vi "Destroy.vi"(8 "ErrorIn":errorcluster, 11 "ReferenceIn":refnum<class "VerticalButtonBar.lvclass">) -> (0 "ErrorOut":errorcluster, 3 "ReferenceOut":refnum<class "VerticalButtonBar.lvclass">)   [LabVIEW 2021, in "VerticalButtonBar.lvclass"]
doc: "Destroy the object instance"
uses:
  VerticalButtonBar.lvclass
  .Externals/Library_TAF_ApplicationFramework/TAFBaseGUI/TAFBaseGUI.lvclass
  VerticalButtonBar.lvclass/VerticalButtonBar.ctl
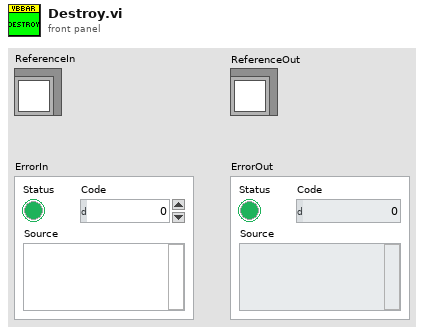
[diagram p1: front panel]
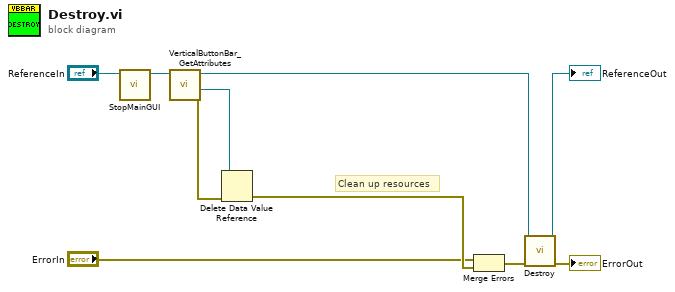
[diagram p0: block diagram]
diagram:
  # "Clean up resources"
  n1 = call "StopMainGUI.vi"("ReferenceIn"="ReferenceIn") -> ("ReferenceOut"=w3:refnum<class "VerticalButtonBar.lvclass">)  [unwired: 9 in, 1 out]
  n2 = call "VerticalButtonBar_GetAttributes.vi"("ReferenceIn"=w3) -> ("ErrorOut"=w10:errorcluster, "DataRef"=w5:refnum<data-value>, "ReferenceOut"=w2:refnum<class "VerticalButtonBar.lvclass">)  [unwired: 7 in, 1 out]
  n3 = Delete Data Value Reference(data value reference=w5, error in=w10) -> (error out=w9:errorcluster)  [unwired: 1 out]
  n4 = Merge Errors("ErrorIn", w9) -> (w7:errorcluster)
  n5 = call-parent "Destroy.vi"("ErrorIn"=w7, "ReferenceIn"=w2) -> ("ErrorOut"=→"ErrorOut":errorcluster, "ReferenceOut"=→"ReferenceOut":refnum<class "VerticalButtonBar.lvclass">)  [unwired: 8 in]
